vi "PFI-28000-Card_Get Frame.vi"(8 "error in (no error)":errorcluster, 11 "PFI-28000-Card in":refnum<class "PFI-28000-Card.lvclass">) -> (0 "error out":errorcluster, 2 "Frame":i32, 3 "PFI-28000-Card out":refnum<class "PFI-28000-Card.lvclass">)   [LabVIEW 2017, in "PFI-28000-Card.lvclass"]
uses:
  PFI-28000-Card.lvclass
  PFI-28000-Card.lvclass/PFI-28000-Card.ctl
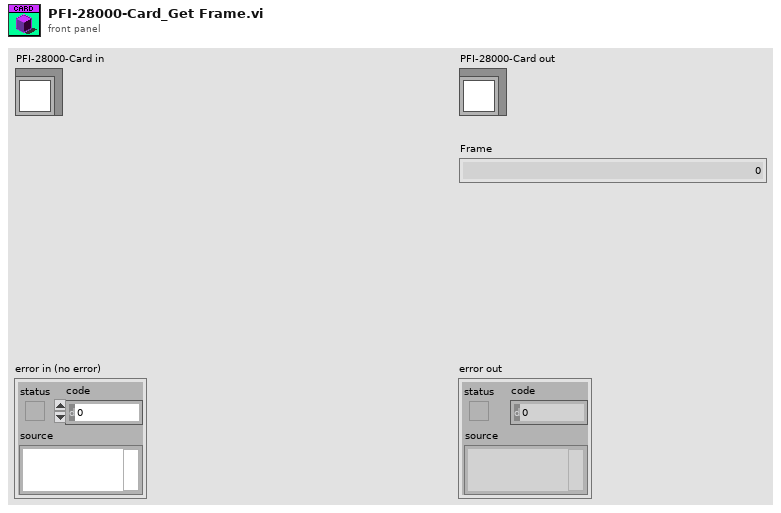
[diagram p1: front panel]
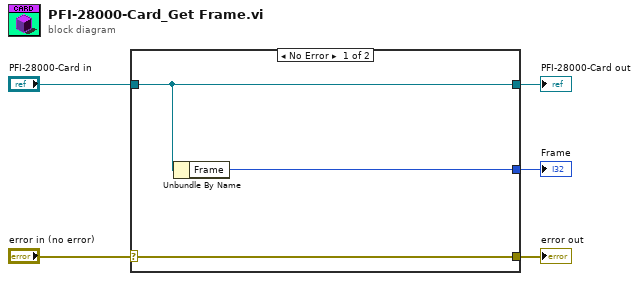
[diagram p0: block diagram]
diagram:
  n1 = case shown="No Error" "error in (no error)" {
    selector: "error in (no error)" -> [w8 w9]
    tunnel: [w8 w9] -> w4
    tunnel: [w7 w10] -> w2
    tunnel: "PFI-28000-Card in" -> [w7 w10]
    tunnel: [w6 _] -> w1
    frame No Error {
      n2 = Unbundle By Name(w7) -> ("Frame"=w6:i32)
    }
    frame Error {
    }
  }
  "error out" <- w4
  "PFI-28000-Card out" <- w2
  "Frame" <- w1
